vi "Call Command.vi"(11 "Command":cluster{"Time (s)":dbl, T1, bool}) -> ()   [LabVIEW 2019]
uses:
  Support Code/Single Cmd Info.ctl
  <vilib>/picture/picture.llb/imagedata.ctl
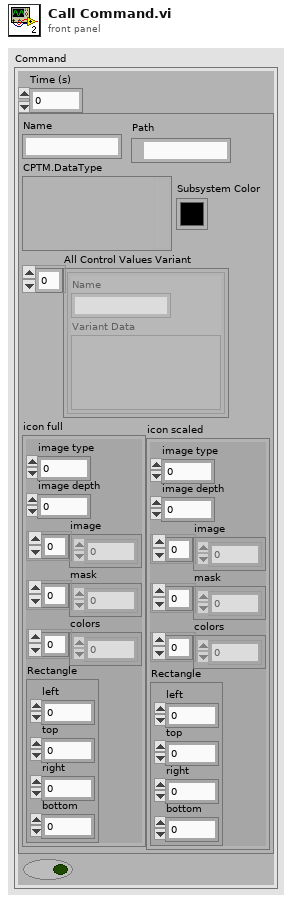
[diagram p1: front panel]
types:
  T1 = typedef "Single Cmd Info.ctl" = cluster{"Name":string, "CPTM.DataType":variant, "All Control Values Variant":cluster{"Name":string, "Variant Data":variant}[], "icon full":T2, "icon scaled":T2, "Path":path, "Subsystem Color":u32}
  T2 = typedef "imagedata.ctl" = cluster{"image type":i32, "image depth":i32, "image":u8[], "mask":u8[], "colors":u32[], "Rectangle":cluster{"left":i16, "top":i16, "right":i16, "bottom":i16}}
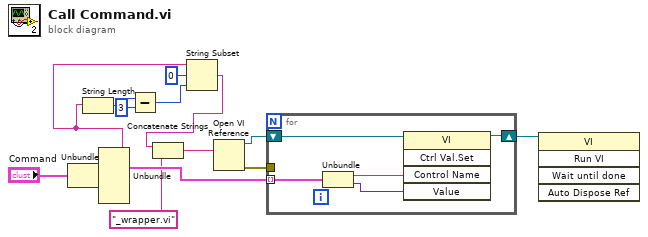
[diagram p0: block diagram]
diagram:
  n1 = Unbundle("Command") -> (w10:T1)  [unwired: 2 out]
  n2 = Unbundle(w10) -> ("Name"=w5:string, "All Control Values Variant"=w9:cluster{"Name":string, "Variant Data":variant}[])  [unwired: 5 out]
  n3 = String Length(string=w5) -> (length=w4:i32)
  n4 = Subtract(x=w4, y=3) -> (x-y=w2:i32)
  n5 = String Subset(string=w5, offset (0)=0, length (rest)=w2) -> (substring=w1:string)
  n6 = Concatenate Strings(w1, "_wrapper.vi" ("string")) -> (w7:string)
  n7 = Open VI Reference(vi path=w7) -> (vi reference=w14:refnum<vi>, error out=w12:errorcluster)  [unwired: 5 in]
  n8 = for {
    tunnel: w9 -> [w19] mode=indexing
    shift-right: [w16] -> w13
    shift-left: w14 -> [w15]
    tunnel: w12 -> [_]
    n9 = Unbundle(w19) -> ("Name"=w18:string, "Variant Data"=w17:variant)
    n10 = invoke class="VI" method="Ctrl Val.Set"(reference=w15, "Control Name"=w18, "Value"=w17) -> (reference out=w16:refnum<vi>)  [unwired: 2 in, 4 out]
  }
  n11 = invoke class="VI" method="Run VI"(reference=w13) -> ()  [unwired: 4 in, 5 out]
